vi "1.6 条码识别.vi"() -> ()   [LabVIEW 2018]
uses:
  <vilib>/vision/Instrument.llb/Barcode Search Options.ctl
  <vilib>/vision/NI_Vision_Development_Module.lvlib
panel:
  out "Image 2":T1(plugin-control)
  out "Barcodes (Barcode Reader 1)":T2(array[cluster]) {"Confidence Level" format="%.2f"; "Barcode Type" items=["Reserved", "Codabar", "Code 39", "Code 93", "Code 128", "EAN 8", "EAN 13", "Interleaved 2 of 5", "MSI", "UPCA", "Pharmacode", "RSS Limited"]; "Bounding Box"."y" format="%.2f"; "Bounding Box"."x" format="%.2f"}
  out "Barcodes":T2(array[cluster]) {"Confidence Level" format="%.2f"; "Barcode Type" items=["Reserved", "Codabar", "Code 39", "Code 93", "Code 128", "EAN 8", "EAN 13", "Interleaved 2 of 5", "MSI", "UPCA", "Pharmacode", "RSS Limited"]; "Bounding Box"."y" format="%.2f"; "Bounding Box"."x" format="%.2f"}
  out "Image":T1(plugin-control)
  in  "File Path":path
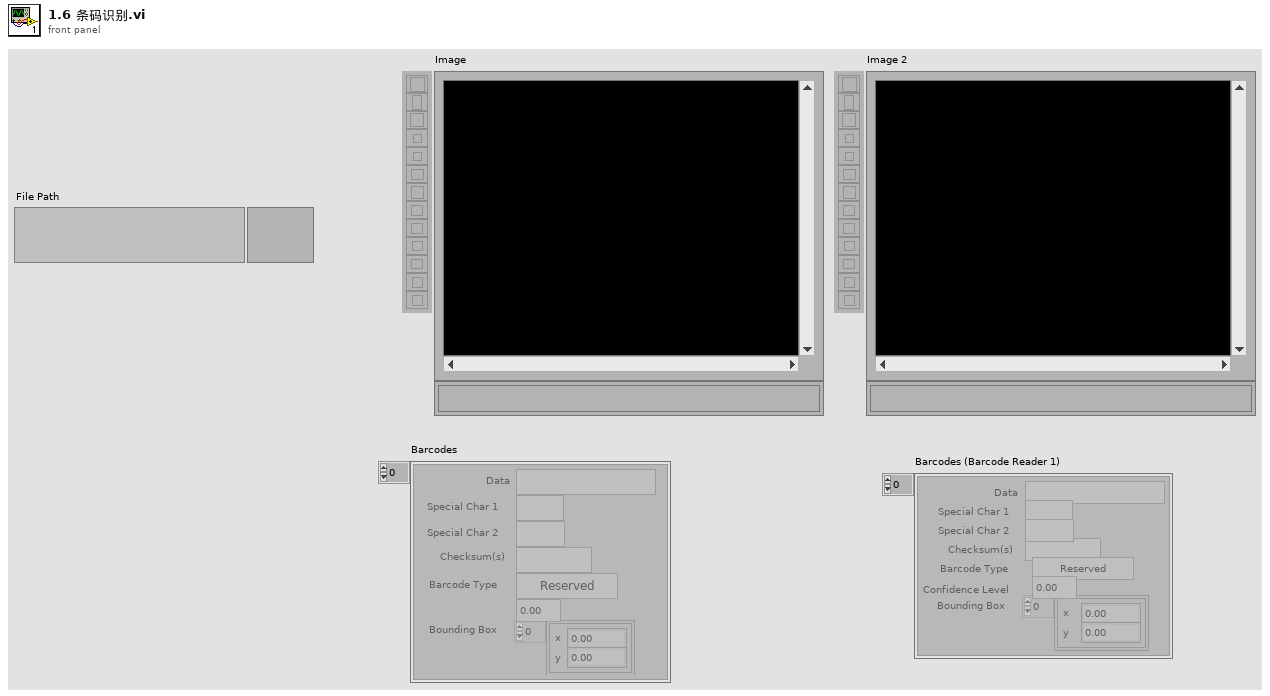
[diagram p1: front panel]
types:
  T1 = typedef "IMAQ Image.ctl" = refnum<image>
  T2 = cluster{"Data":string, "Special Char 1":string, "Special Char 2":string, "Checksum(s)":string, "Barcode Type":u32, "Confidence Level":sgl, "Bounding Box":cluster{"x":sgl, "y":sgl}[]}[]
  T3 = cluster{"Brightness":sgl, "Contrast":sgl, "Gamma":sgl}
  T4 = typedef "Barcode Search Options.ctl" = cluster{"Min Bar Width":u32, "Min Edge Strength":u32, "Min Bars":u32, "Skip Location Search?":bool}
  T5 = typedef "Image Type" = u32
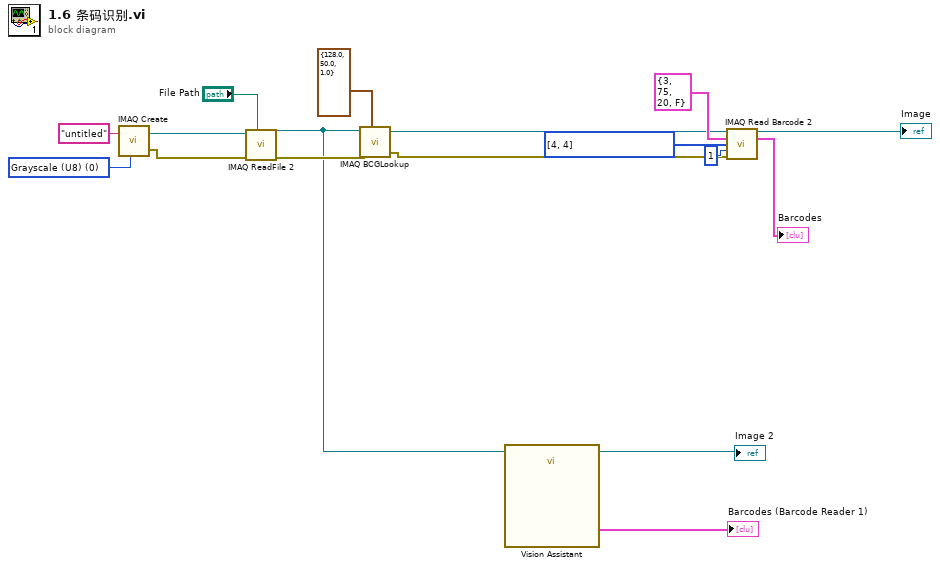
[diagram p0: block diagram]
diagram:
  w11 = u32[] [4, 4] items=["Reserved", "Codabar", "Code 39", "Code 93", "Code 128", "EAN 8", "EAN 13", "Interleaved 2 of 5", "MSI", "UPCA", "Pharmacode", "RSS Limited"] ("Barcode Types To Search")
  w16 = T5 0 items=["Grayscale (U8)", "Grayscale (I16)", "Grayscale (SGL)", "Complex (CSG)", "RGB (U32)", "HSL (U32)", "RGB (U64)", "Grayscale (U16)"] ("Image Type")
  n1 = call "IMAQ Create"("Image Name"="untitled", "Image Type"=w16) -> ("New Image"=w15:T1, "error out"=w14:errorcluster)  [unwired: 3 in]
  n2 = call "IMAQ ReadFile 2"("File Path"="File Path", "error in (no error)"=w14, "Image"=w15) -> ("error out"=w5:errorcluster, "Image Out"=w2:T1)  [unwired: 4 in, 3 out]
  n3 = call "IMAQ BCGLookup"("Image Src"=w2, "BCG Values"=T3 {"Brightness"=128.0, "Contrast"=50.0, "Gamma"=1.0}, "error in (no error)"=w5) -> ("Image Dst Out"=w7:T1, "error out"=w4:errorcluster)  [unwired: 4 in]
  n4 = call "Vision Assistant"("Image In"=w2) -> ("Image Out"=→"Image 2":T1, "Barcodes (Barcode Reader 1)"=→"Barcodes (Barcode Reader 1)":T2)  [unwired: 24 in, 1 out]
  n5 = call "IMAQ Read Barcode 2"("Image"=w7, "Barcode Search Options"=T4 {"Min Bar Width"=3, "Min Edge Strength"=75, "Min Bars"=20, "Skip Location Search?"=FALSE}, "Barcode Types To Search"=w11, "Num of Required Barcodes"=u32 1, "error in (no error)"=w4) -> ("Image (duplicate)"=→"Image":T1, "Barcodes"=→"Barcodes":T2)  [unwired: 6 in, 3 out]
